vi "Input Register Set Mapping.vi"(8 "error in (no error)":errorcluster, 10 "Mapping":T2, 11 "Item Ref in":T1 format="%.0x") -> (0 "error out":errorcluster, 3 "Item Ref out":T1 format="%.0x")   [LabVIEW 2015, in "Modbus Master System Explorer.lvlib"]
uses:
  Modbus Master System Explorer.lvlib
  <vilib>/NI Veristand/Custom Device API/Custom Device Item Ref.ctl
  Shared/Controls/Data Model/Mapping.ctl
  Shared/Controls/Data Model/DataType.ctl
  <vilib>/NI VeriStand/Custom Device API/Custom Device API.lvlib
  Shared/Modbus Master Shared.lvlib
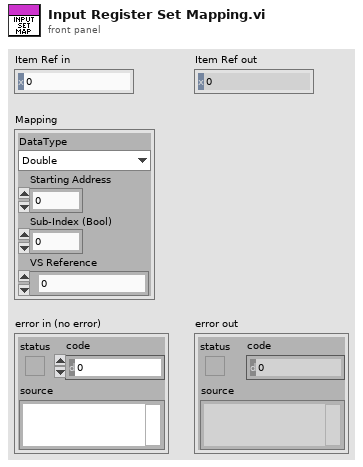
[diagram p1: front panel]
types:
  T1 = typedef "Custom Device API.lvlib/Custom Device Item Ref.ctl" = u64
  T2 = typedef "Modbus Master Shared.lvlib/Mapping.ctl" = cluster{"DataType":T3, "Starting Address":u16, "Sub-Index (Bool)":u16, "VS Reference":T1}
  T3 = typedef "Modbus Master Shared.lvlib/DataType.ctl" = enum16{"Double", "Single", "I64", "I32", "I16", "I8", "U64", "U32", "U16", "U8", "Boolean"}
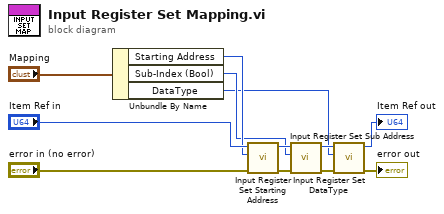
[diagram p0: block diagram]
diagram:
  n1 = Unbundle By Name("Mapping") -> ("Starting Address"=w3:u16, "Sub-Index (Bool)"=w2:u16, "DataType"=w1:T3)
  n2 = call "Input Register Set Starting Address.vi"("error in (no error)"="error in (no error)", "Value"=w3, "Item Ref in"="Item Ref in") -> ("error out"=w10:errorcluster, "Item Ref out"=w11:T1)  [unwired: 7 in]
  n3 = call "Input Register Set Sub Address.vi"("error in (no error)"=w10, "Value"=w2, "Item Ref in"=w11) -> ("error out"=w8:errorcluster, "Item Ref out"=w9:T1)  [unwired: 7 in]
  n4 = call "Input Register Set DataType.vi"("error in (no error)"=w8, "DataType"=w1, "Item Ref in"=w9) -> ("error out"=→"error out":errorcluster, "Item Ref out"=→"Item Ref out":T1)  [unwired: 7 in]
